vi "Temp.vi"() -> ()   [LabVIEW 2019]
uses:
  <vilib>/Simulation/Scripting/Companion Diagram/SimConfigNode/SimParams.ctl
  <vilib>/Simulation/Scripting/Companion Diagram/SimConfigNode/_simSolvers.ctl
  <vilib>/Simulation/Implementation/Shared/SIMSCR Execution Mode.ctl
  <vilib>/Simulation/Param Hierarchy/Typedefs/SIMPH Param Control Actions.ctl
  <vilib>/addons/System Identification/Model Typedefs.llb/SI Model Type.ctl
  <vilib>/Analysis/1siggen.llb/Ramp Pattern by Samples.vi
  <vilib>/Simulation/Implementation/Shared/NILVSim_ParamChanged.vi
  <vilib>/Simulation/Implementation/Shared/NILVSIM_BeginStep.vi
  <vilib>/Simulation/DataSources/Implementation/NILVSim Chirp Signal.llb/SIM Chirp Signal (scalar).vi
  <vilib>/Simulation/Utility/Implementation/SIM Halt.vi
  <vilib>/Simulation/Utility/Implementation/NILVSim Indexer (Imp).llb/SIM Index by Time (Waveform).vi
  <vilib>/Simulation/Utility/Implementation/SIM Time.vi
  <vilib>/Simulation/LookUpTables/Implementation/NILVSim LUT 1D.llb/SIM LUT 1D (scalar).vi
  <vilib>/Simulation/SignalDisplay/Implementation/NILVSim Time Waveform.llb/SIM Time Waveform (vector).vi
  <vilib>/Simulation/Implementation/Shared/NILVSim_Manager.vi
  <vilib>/Utility/error.llb/Clear Errors.vi
  <vilib>/Simulation/Implementation/Shared/NILVSim_FinalizeModel.vi
  <vilib>/Simulation/Utility/Implementation/NILVSim Indexer (Imp).llb/NILVSim Index by Time Core (Waveform).vi
  <vilib>/Simulation/Implementation/Shared/SIM Interpolate.llb/SIM Interpolate (Waveform).vi
  <vilib>/Simulation/Implementation/Shared/SIM Interpolate.llb/SIM Interpolate (array).vi
  <vilib>/Simulation/Implementation/Shared/SIM Unbundle Sim Info.vi
  <vilib>/Simulation/Implementation/Shared/NILVSim_Initialize.vi
  <vilib>/addons/System Identification/Model Management.llb/SI Create System Model.vi
  <vilib>/addons/System Identification/Model Presentation.llb/SI Bode Plot.vi
  <vilib>/Simulation/Utility/Implementation/NILVSim Get Time and IsAcceptedStep.vi
  <vilib>/addons/System Identification/Data Preprocess.llb/SI Lowpass Filter.vi
  <vilib>/addons/System Identification/Data Preprocess.llb/SI Lowpass Filter (MISO Waveform).vi
  <vilib>/Simulation/Implementation/Shared/SIMSH Read Queue.vi
  <vilib>/Simulation/Implementation/Shared/NILVSim_GetModelError.vi
  <vilib>/Simulation/Implementation/Shared/SIM Bundle Sim Info.vi
  <vilib>/Simulation/Scripting/Companion Diagram/SimConfigNode/SimDog.xnode
  <vilib>/Simulation/Implementation/XNodeFramework/SimXNode/SimX.xnode
  <vilib>/Analysis/NI_AALBase.lvlib
  <vilib>/addons/System Identification/NI_SysID.lvlib
  <vilib>/Simulation/Implementation/Shared/NI_SIM_Implementation.lvlib
panel:
  in  "target frequency":dbl=3.0
  in  "target time":dbl=10.0
  in  "initial frequency":dbl=0.01
  in  "stop":bool
  out "Waveform Chart":waveform(dbl)[](graph)=[{"t0"=timestamp(20 s since 1904-01-01), "dt"=1.0, "Y"=[0.0]}, {"t0"=timestamp(20 s since 1904-01-01), "dt"=1.0, "Y"=[0.12542642593691802]}, {"t0"=timestamp(20 s since 1904-01-01), "dt"=1.0, "Y"=[0.0]}]
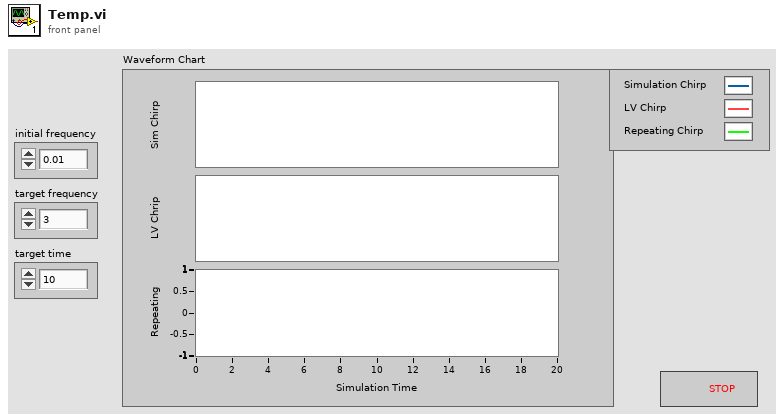
[diagram p1: front panel]
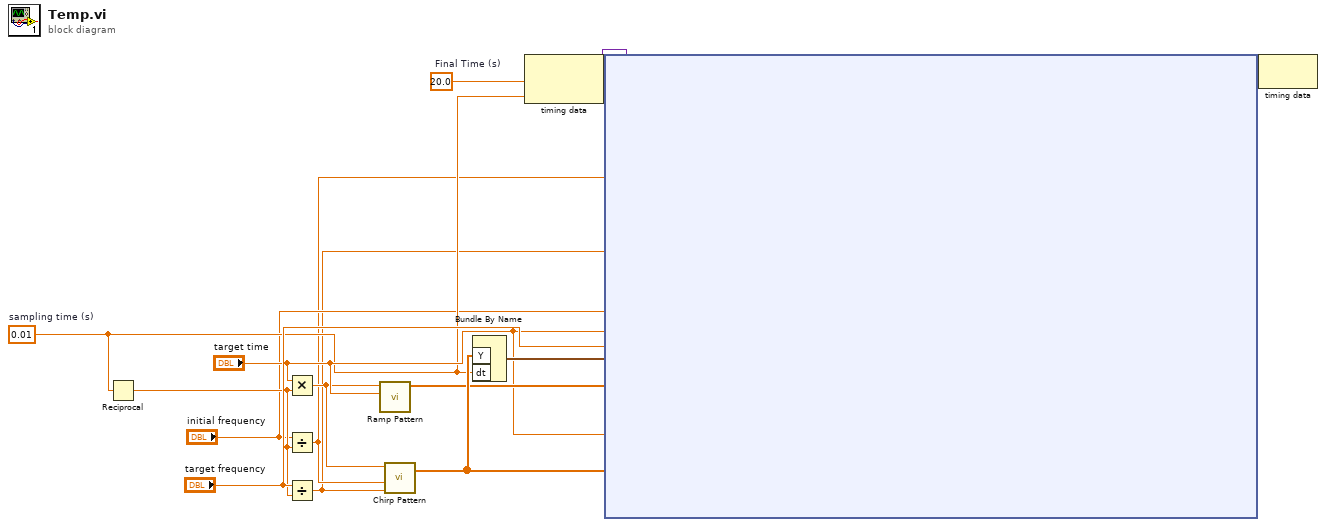
[diagram p0: block diagram]
diagram:
  w10 = 20.0  # Final Time (s)
  w6 = 0.01  # sampling time (s)
  n1 = Reciprocal(x=w6) -> (1/x=w5:dbl)
  n2 = Multiply(x="target time", y=w5) -> (x*y=w4:dbl)
  n3 = Divide(x="initial frequency", y=w5) -> (x/y=w2:dbl)
  n4 = Divide(x="target frequency", y=w5) -> (x/y=w1:dbl)
  n5 = call-poly <vilib>:"Ramp Pattern.vi"("end"="target time", "samples"=w4) -> ("Ramp Pattern"=w8:dbl[])  [unwired: 8 in, 1 out]
  n6 = call <vilib>:"Chirp Pattern.vi"("f2"=w1, "f1"=w2, "samples"=w4) -> ("Chirp Pattern"=w9:dbl[])  [unwired: 1 in, 1 out]
  n7 = Bundle By Name("Y"=w9, "dt"=w6) -> (w12:waveform(dbl))  [unwired: 1 in]
  n8 = node-c288(w10, w6) -> (w14:variant)
  n9 = node-c254 ("Control & Simulation Loop")(w14, w12, "initial frequency", "target time", "target frequency", w9, w8, "target time", w2, w1) -> (w13:variant)
  n10 = node-c288(w13) -> ()  [unwired: 1 out]
